vi "2 Arithmetic.vi"() -> ()   [LabVIEW 2015]
panel:
  in  "y":dbl
  in  "x":dbl
  out "z":dbl
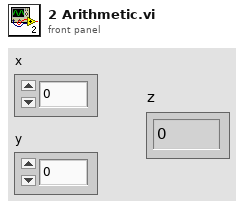
[diagram p1: front panel]
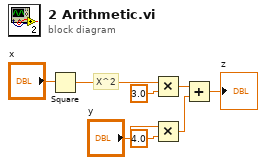
[diagram p0: block diagram]
diagram:
  # "X^2"
  n1 = Square(x="x") -> (x^2=w7:dbl)
  n2 = Multiply(x=w7, y=3.0) -> (x*y=w5:dbl)
  n3 = Multiply(x="y", y=4.0) -> (x*y=w2:dbl)
  n4 = Add(x=w5, y=w2) -> (x+y=→"z":dbl)
